vi "LeerRutaBaseDeDatos.vi"(8 "error in (no error)":errorcluster) -> (0 "error out":errorcluster, 2 "Database Path":path)   [LabVIEW 2019, in "Base de Datos.lvclass"]
uses:
  Base de Datos.lvclass
  <vilib>/Utility/config.llb/Read Key (String).vi
  <vilib>/Utility/config.llb/NI_LVConfig.lvlib
panel:
  out "DB out":refnum<class "Base de Datos.lvclass">
  out "RutaBD":string
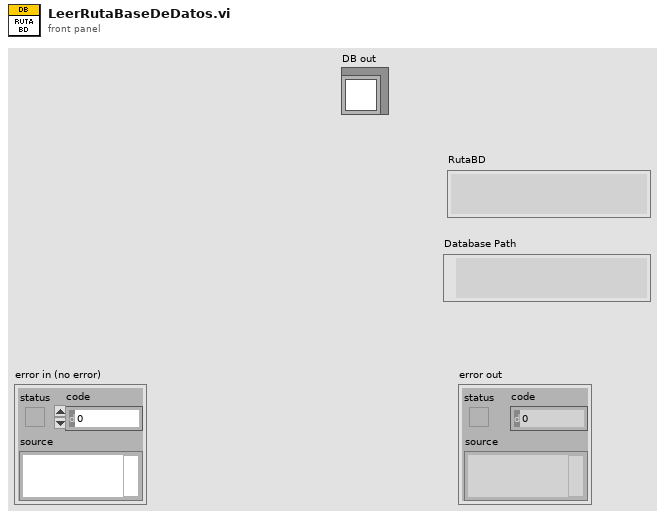
[diagram p1: front panel]
types:
  T1 = typedef "NI_LVConfig.lvlib/Config Data RefNum.ctl" = refnum<k1>
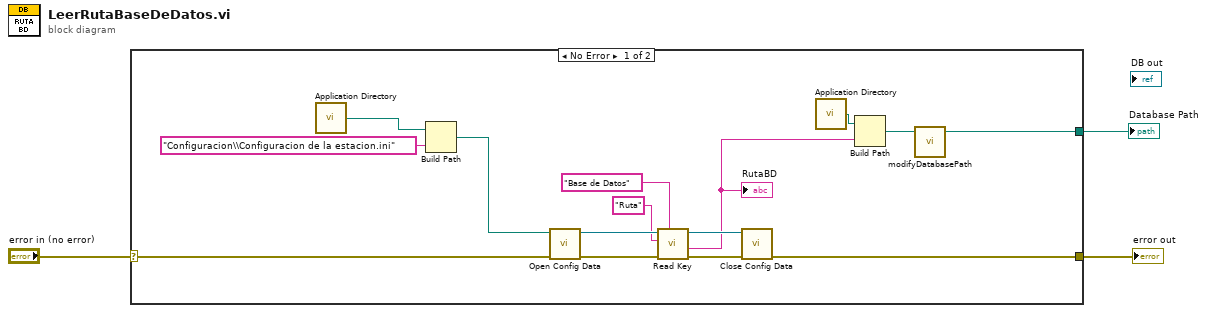
[diagram p0: block diagram]
diagram:
  n1 = case shown="No Error" "error in (no error)" {
    selector: "error in (no error)" -> [w9 w19]
    tunnel: [w4 w19] -> w2
    tunnel: [w5 _] -> w1
    frame No Error {
      n2 = call <vilib>:"Application Directory.vi"() -> ("Application Directory"=w17:path)
      n3 = Build Path(base path=w17, name or relative path="Configuracion\\Configuracion de la estacion.ini") -> (appended path=w10:path)
      n4 = call <vilib>:"Open Config Data.vi"("error in (no error)"=w9, "configuration file path"=w10) -> ("error out"=w16:errorcluster, "refnum"=w15:T1)  [unwired: 7 in, 1 out]
      n5 = call-poly <vilib>:"Read Key.vi"("section"="Base de Datos", "error in (no error)"=w16, "key"="Ruta", "refnum"=w15) -> ("error out"=w14:errorcluster, "value"=w6:string, "refnum out"=w13:T1)  [unwired: 4 in, 1 out]
      "RutaBD" <- w6
      n6 = call <vilib>:"Close Config Data.vi"("error in (no error)"=w14, "refnum"=w13) -> ("error out"=w4:errorcluster)  [unwired: 8 in, 1 out]
      n7 = call <vilib>:"Application Directory.vi"() -> ("Application Directory"=w8:path)
      n8 = Build Path(base path=w8, name or relative path=w6) -> (appended path=w7:path)
      n9 = call "modifyDatabasePath.vi"("Database Path In"=w7) -> ("Database Path Out"=w5:path)  [unwired: 4 in]
    }
    frame Error {
    }
  }
  "error out" <- w2
  "Database Path" <- w1
